vi "WriteTransducer.vi"(0 "sensor":T1(array[cluster]), 1 "file path":path) -> ()   [LabVIEW 2011]
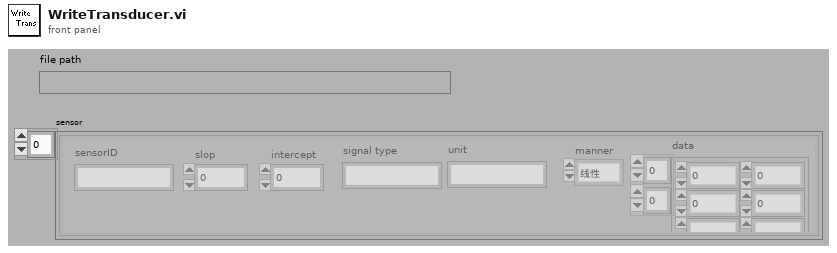
[diagram p1: front panel]
types:
  T1 = cluster{"manner":enum16{"线性", "查表"}, "data":dbl[][], "slop":dbl, "intercept":dbl, "sensorID":string, "signal type":string, "unit":string}[]
  T2 = enum16{"big-endian, network order", "native, host order", "little-endian"}
  T3 = enum16{"open", "replace", "create", "open or create", "replace or create", "replace or create with confirmation"}
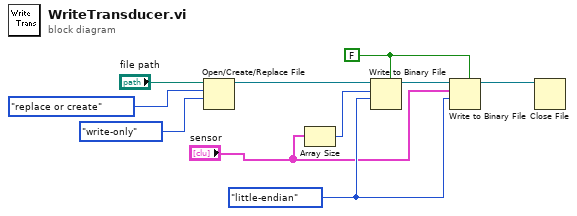
[diagram p0: block diagram]
diagram:
  w3 = T2."little-endian" ("byte order (0:big-endian, network order)")
  w4 = FALSE ("prepend array or string size? (T)")
  n1 = Open/Create/Replace File(file path (use dialog)="file path", operation (0:open)=T3."replace or create", access (0:read/write)=enum16{"read/write", "read-only", "write-only"}."write-only") -> (refnum out=w7:refnum<file>)  [unwired: 1 in, 4 out]
  n2 = Array Size(array="sensor") -> (size(s)=w6:i32)
  n3 = Write to Binary File(file (use dialog)=w7, data=w6, 5:w4, 9:w3) -> (refnum out=w5:refnum<file>)  [unwired: 1 in, 3 out]
  n4 = Write to Binary File(file (use dialog)=w5, data="sensor", 5:w4, 9:w3) -> (refnum out=w2:refnum<file>)  [unwired: 1 in, 3 out]
  n5 = Close File(refnum=w2) -> ()  [unwired: 1 in, 2 out]
